vi "Remove RTs.vi"(8 "error in":errorcluster, 11 "Target in":refnum<k24>) -> (0 "error out":errorcluster, 3 "Target out":refnum<k24>)   [LabVIEW 2020]
uses:
  NationalInstruments.VeriStand.SystemDefinitionAPI
  Scripting/AIM MIL-STD-1553 Scripting.lvlib
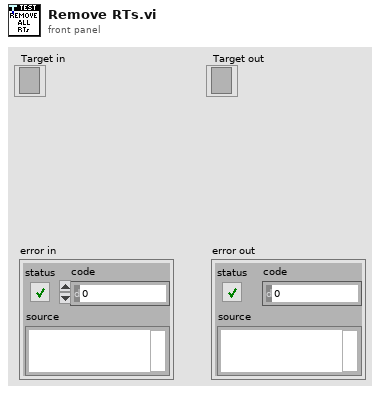
[diagram p1: front panel]
types:
  T1 = typedef "Custom Device API.lvlib/Custom Device Item Ref.ctl" = u64
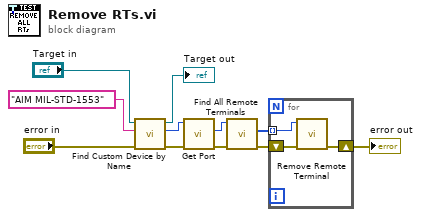
[diagram p0: block diagram]
diagram:
  n1 = call "Find Custom Device by Name.vi"("error in"="error in", "custom device name"="AIM MIL-STD-1553" ("name"), "target"="Target in") -> ("error out"=w6:errorcluster, "custom device"=w5:T1, "target out"=→"Target out":refnum<k24>)  [unwired: 5 in, 1 out]
  n2 = call "Get Port.vi"("error in"=w6, "custom device ref"=w5) -> ("error out"=w8:errorcluster, "port"=w7:T1)  [unwired: 6 in, 2 out]
  n3 = call "Find All Remote Terminals.vi"("error in"=w8, "port"=w7) -> ("error out"=w10:errorcluster, "remote terminals"=w9:T1[])  [unwired: 7 in, 1 out]
  n4 = for {
    tunnel: w9 -> [w14] mode=indexing
    shift-right: [w12] -> w11
    shift-left: w10 -> [w13]
    n5 = call "Remove Remote Terminal.vi"("error in"=w13, "remote terminal"=w14) -> ("error out"=w12:errorcluster)  [unwired: 9 in]
  }
  "error out" <- w11
